vi "ex1_call_collect.vi"() -> ()   [LabVIEW 2022 SP3]
uses:
  pylabview/pythonq.lvlib
  C:/Program Files (x86)/National Instruments/LabVIEW 2022/examples/Connectivity/Python/support/PythonVersionsEnum.ctl
  py_msg.ctl
panel:
  in  "start at":i32
  out "l2":bool
  out "l1":bool
  in  "data_points":i32=100
  out "Numeric 2":i32
  out "Numeric 1":i32
  out "count 2":i32
  out "count":i32
  out "er_data_in":errorcluster
  out "er_count":errorcluster
  out "er_end":errorcluster
  out "Waveform Graph":dbl[](graph)
  # "# Created by Jeff Morgan\n# https://awakeniot.com/"
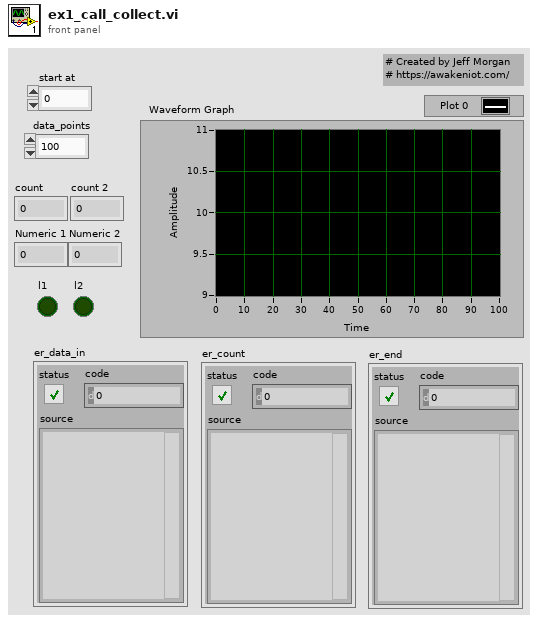
[diagram p1: front panel]
types:
  T1 = typedef "PythonVersionsEnum.ctl" = enum16{"3.6", "3.7", "3.8", "3.9"}
  T2 = typedef "pythonq.lvlib/py_cluster.ctl" = cluster{"path":path, "py":T3}
  T3 = typedef "pythonq.lvlib/py_session.ctl" = cluster{"session":refnum<k35>, "object":refnum<k38>}
  T4 = typedef "py_msg.ctl" = cluster{"double":dbl, "ref":string}
  T5 = typedef "pythonq.lvlib/py_result.ctl" = cluster{"value":string, "ok":bool, "error_msg":string}
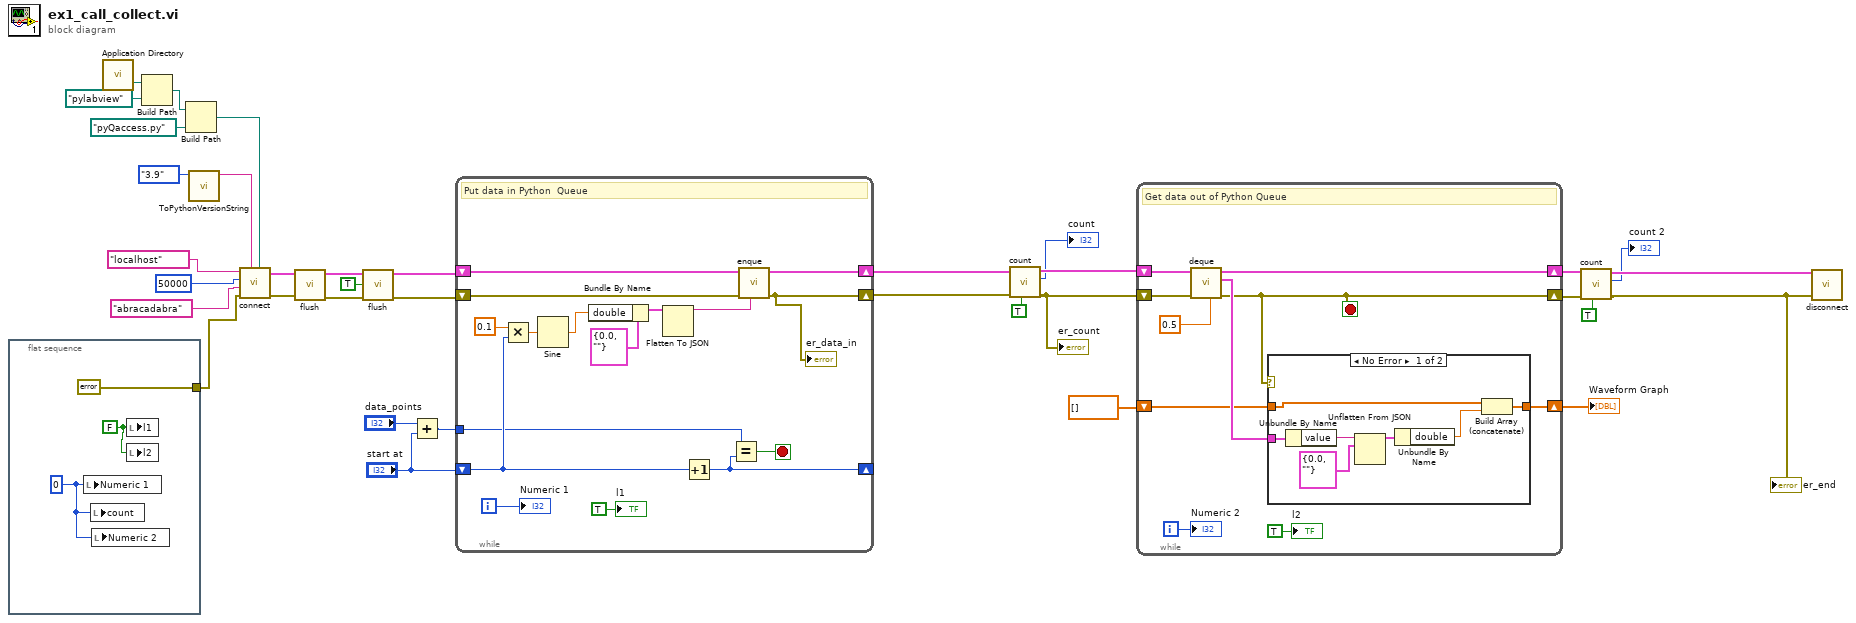
[diagram p0: block diagram]
diagram:
  n1 = flat-sequence {
    tunnel: [errorcluster {"status"=FALSE, "code"=0, "source"=""} ("error in (no error)")] -> w14
    frame #0 {
      w37 = 0 ("Numeric")
      w38 = FALSE ("l1")
      n2 = local write "Numeric 1"(w37) -> ()
      n3 = local write "count"(w37) -> ()
      n4 = local write "Numeric 2"(w37) -> ()
      n5 = local write "l1"(w38) -> ()
      n6 = local write "l2"(w38) -> ()
    }
  }
  n7 = call <vilib>:"Application Directory.vi"() -> ("Application Directory"=w30:path)
  n8 = Build Path(base path=w30, name or relative path=path "pylabview") -> (appended path=w31:path)
  n9 = Build Path(base path=w31, name or relative path=path "pyQaccess.py") -> (appended path=w28:path)
  n10 = call "ToPythonVersionString.vi"("python version"=PythonVersionsEnum."3.9") -> ("python version string"=w33:string)  [unwired: 10 in]
  n11 = call "connect.vi"("module path"=w28, "Python version"=w33, "error in (no error)"=w14, "password"="abracadabra", "port"=50000, "ip_address"="localhost") -> ("error out"=w17:errorcluster, "py out"=w18:T2)  [unwired: 4 in]
  n12 = call "flush.vi"("error in (no error)"=w17, "py in"=w18) -> ("error out"=w8:errorcluster, "py out"=w7:T2)  [unwired: 8 in]
  n13 = call "flush.vi"("error in (no error)"=w8, "out?"=TRUE, "py in"=w7) -> ("error out"=w6:errorcluster, "py out"=w5:T2)  [unwired: 7 in]
  n14 = Add(x="data_points", y="start at") -> (x+y=w1:i32)
  n15 = while {
    shift-right: [w53] -> w10
    shift-left: w6 -> [w54]
    shift-right: [w52] -> w11
    shift-left: w5 -> [w51]
    shift-right: [w50] -> _
    shift-left: "start at" -> [w42]
    tunnel: w1 -> [w39]
    i -> [w49]
    stop <- w48 stop-if-true
    # "Put data in Python  Queue"
    n16 = Multiply(x=0.1, y=w42) -> (x*y=w40:dbl)
    n17 = Sine(x=w40) -> (sin(x)=w43:dbl)
    n18 = Bundle By Name(cluster=T4 {"double"=0.0, "ref"=""} ("Cluster"), "double"=w43) -> (w47:T4)
    n19 = Flatten To JSON(anything=w47) -> (JSON string=w45:string)  [unwired: 2 in, 1 out]
    n20 = Increment(x=w42) -> (x+1=w50:i32)
    n21 = Equal?(x=w39, y=w50) -> (x = y?=w48:bool)
    n22 = call "enque.vi"("data in"=w45, "error in (no error)"=w54, "py in"=w51) -> ("error out"=w53:errorcluster, "py out"=w52:T2)  [unwired: 5 in, 2 out]
    "er_data_in" <- w53
    "Numeric 1" <- w49
    "l1" <- TRUE ("l1")
  }
  n23 = call "count.vi"("quein?"=TRUE, "error in (no error)"=w10, "py in"=w11) -> ("error out"=w26:errorcluster, "count"=→"count":i32, "py out"=w25:T2)  [unwired: 6 in]
  "er_count" <- w26
  n24 = while {
    shift-right: [w62] -> w22
    shift-left: w25 -> [w63]
    shift-right: [w59] -> w23
    shift-left: w26 -> [w64]
    shift-right: [w58] -> w16
    shift-left: dbl[] [] -> [w57]
    i -> [w61]
    stop <- w59 stop-if-true
    # "Get data out of Python Queue"
    n25 = call "deque.vi"("timeout"=0.5, "error in (no error)"=w64, "py in"=w63) -> ("error out"=w59:errorcluster, "response"=w60:T5, "py out"=w62:T2)  [unwired: 5 in, 1 out]
    n26 = case shown="No Error" w59 {
      tunnel: w60 -> [w69 _]
      tunnel: [w66 w72] -> w58
      tunnel: w57 -> [w65 w72]
      frame No Error {
        n27 = Unbundle By Name(w69) -> ("value"=w71:string)
        n28 = Unflatten From JSON(JSON string=w71, type and defaults=T4 {"double"=0.0, "ref"=""} ("Cluster")) -> (value=w68:T4)  [unwired: 5 in, 1 out]
        n29 = Unbundle By Name(w68) -> ("double"=w67:dbl)
        n30 = Build Array (concatenate)(w65, w67) -> (w66:dbl[])
      }
      frame Error {
      }
    }
    "Numeric 2" <- w61
    "l2" <- TRUE ("l2")
  }
  "Waveform Graph" <- w16
  n31 = call "count.vi"("quein?"=TRUE, "error in (no error)"=w23, "py in"=w22) -> ("error out"=w20:errorcluster, "count"=→"count 2":i32, "py out"=w21:T2)  [unwired: 6 in]
  "er_end" <- w20
  n32 = call "disconnect.vi"("error in (no error)"=w20, "py in"=w21) -> ()  [unwired: 9 in, 1 out]
